vi "Configure Waveform (User Defined).vi"(0 "VISA resource name":refnum<visa-resource-name>, 1 "User Defined Level":dbl[](array[numeric]) format="%^.3e", 5 "Channel Name (1)":string="1", 7 "User Defined Beginning Step":bool[](array[boolean]), 9 "Waveform Type (1: Voltage)":i32(ring)=1 items=["Voltage"=1, "Current"=0], 11 "error in (no error)":errorcluster {"code" format="%.0x"}, 12 "User Defined Dwell Time":dbl[](array[numeric]) format="%^.3e") -> (4 "VISA resource name out":refnum<visa-resource-name>, 15 "error out":errorcluster {"code" format="%.0x"})   [LabVIEW 2016, in "Agilent N6700 Series.lvlib"]
doc: "Configures the user defined waveform.\n\n<b>Note:</b>\nThis VI only applies to the N6705B and N6705C DC Power Analyzer."
uses:
  <instrlib>/Agilent N6700 Series/Agilent N6700 Series.lvlib
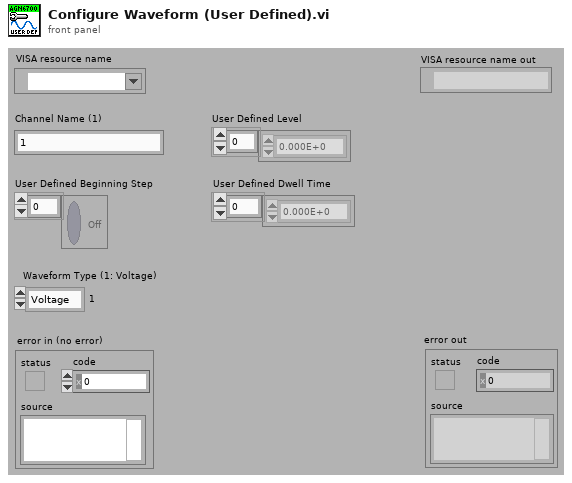
[diagram p1: front panel]
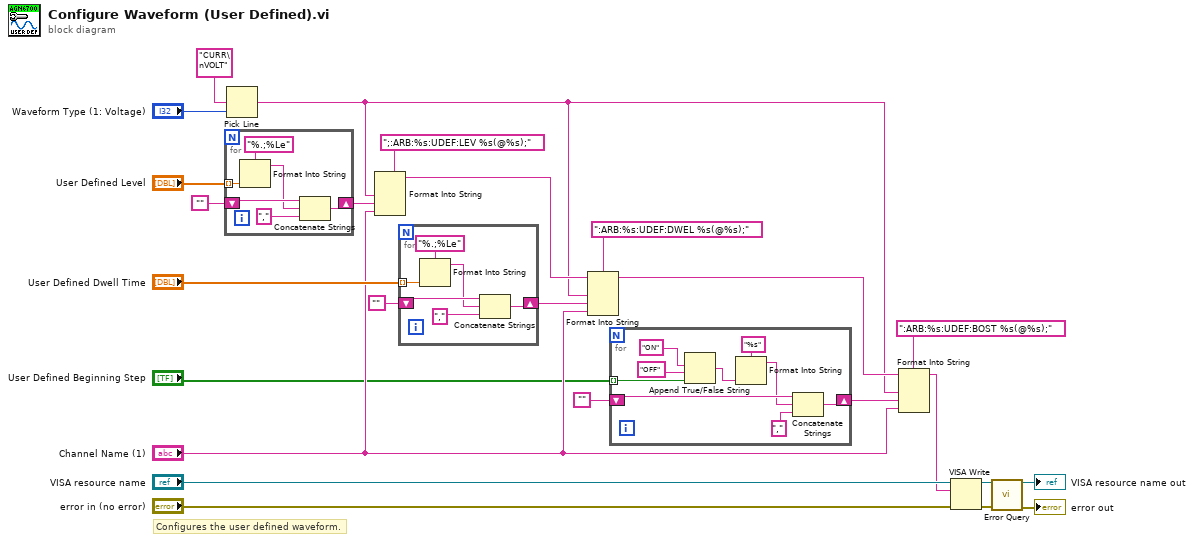
[diagram p0: block diagram]
diagram:
  # "Configures the user defined waveform."
  n1 = for {
    tunnel: "User Defined Level" -> [w27] mode=indexing
    shift-right: [w31] -> w12
    shift-left: "" ("Empty String Constant") -> [w30]
    n2 = Format Into String(format string="%.;%Le", w27) -> (resulting string=w26:string)  [unwired: 2 in, 1 out]
    n3 = Concatenate Strings(w30, w26, ",") -> (w31:string)
  }
  n4 = Pick Line(multi-line string="CURR\nVOLT", line index="Waveform Type (1: Voltage)") -> (output string=w1:string)  [unwired: 1 in]
  n5 = Format Into String(format string=";:ARB:%s:UDEF:LEV %s(@%s);", w1, w12, "Channel Name (1)") -> (resulting string=w5:string)  [unwired: 2 in, 1 out]
  n6 = for {
    tunnel: "User Defined Dwell Time" -> [w33] mode=indexing
    shift-right: [w37] -> w10
    shift-left: "" ("Empty String Constant") -> [w36]
    n7 = Format Into String(format string="%.;%Le", w33) -> (resulting string=w32:string)  [unwired: 2 in, 1 out]
    n8 = Concatenate Strings(w36, w32, ",") -> (w37:string)
  }
  n9 = Format Into String(format string=":ARB:%s:UDEF:DWEL %s(@%s);", initial string=w5, w1, w10, "Channel Name (1)") -> (resulting string=w2:string)  [unwired: 1 in, 1 out]
  n10 = for {
    tunnel: "User Defined Beginning Step" -> [w39] mode=indexing
    shift-right: [w46] -> w4
    shift-left: "" ("Empty String Constant") -> [w45]
    n11 = Append True/False String(1:w39, 2:"OFF", 3:"ON") -> (0:w38:string)  [unwired: 1 in]
    n12 = Format Into String(format string="%s", w38) -> (resulting string=w42:string)  [unwired: 2 in, 1 out]
    n13 = Concatenate Strings(w45, w42, ",") -> (w46:string)
  }
  n14 = Format Into String(format string=":ARB:%s:UDEF:BOST %s(@%s);", initial string=w2, w1, w4, "Channel Name (1)") -> (resulting string=w3:string)  [unwired: 1 in, 1 out]
  n15 = VISA Write(VISA resource name="VISA resource name", write buffer=w3, error in (no error)="error in (no error)") -> (VISA resource name out=w21:refnum<visa-resource-name>, error out=w20:errorcluster)  [unwired: 1 out]
  n16 = call <instrlib>:"Error Query.vi"("VISA resource name"=w21, "error in (no error)"=w20) -> ("VISA resource name out"=→"VISA resource name out":refnum<visa-resource-name>, "error out"=→"error out":errorcluster)  [unwired: 10 in, 2 out]
